vi "HeightPreset.vi"(11 "Height":dbl) -> (3 "Sensor Units":i32)   [LabVIEW 2018]
uses:
  Configuration/Constants.vi
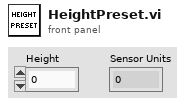
[diagram p1: front panel]
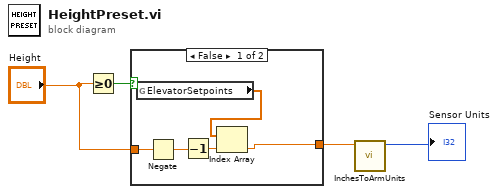
[diagram p0: block diagram]
diagram:
  n1 = Greater Or Equal To 0?(x="Height") -> (x >= 0?=w2:bool)
  n2 = case shown="False" w2 {
    tunnel: "Height" -> [w6 w10]
    tunnel: [w5 w10] -> w3
    frame False {
      n3 = global read "Constants.vi" "ElevatorSetpoints"() -> (w9:dbl[])
      n4 = Negate(x=w6) -> (-x=w8:dbl)
      n5 = Decrement(x=w8) -> (x-1=w7:dbl)
      n6 = Index Array(array=w9, index=w7) -> (element=w5:dbl)
    }
    frame True {
    }
  }
  n7 = call "InchesToArmUnits.vi"("Inches"=w3) -> ("Sensor Units"=→"Sensor Units":i32)  [unwired: 10 in]
